vi "Abort.vi"(8 "error in (no error)":errorcluster, 11 "Parallell Test Runner in":refnum<class "Parallel Test Runner.lvclass">) -> (0 "error out":errorcluster)   [LabVIEW 2020, in "Parallel Test Runner.lvclass"]
uses:
  Parallel Test Runner.lvclass
  Parallel Test Runner.lvclass/Parallel Test Runner.ctl
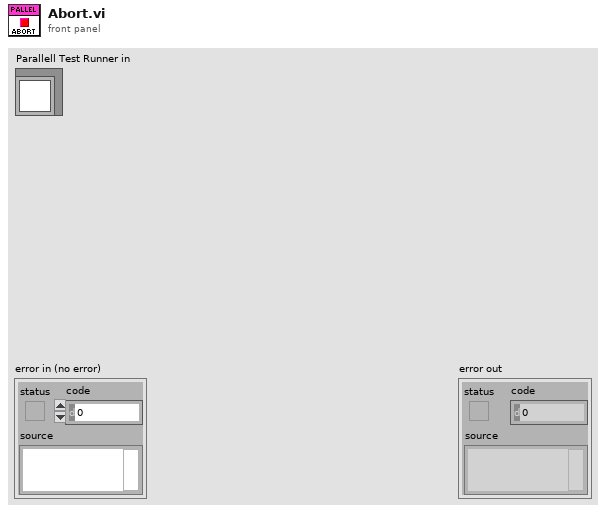
[diagram p1: front panel]
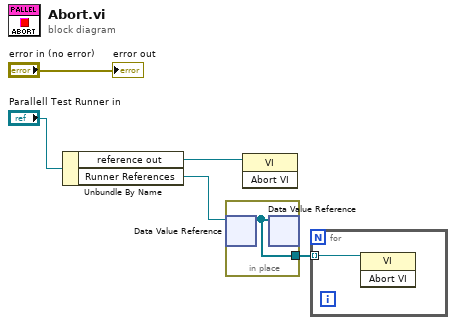
[diagram p0: block diagram]
diagram:
  n1 = Unbundle By Name("Parallell Test Runner in") -> ("reference out"=w3:refnum<vi>, "Runner References"=w2:refnum<data-value>)
  n2 = in-place {
    in-place-border: [w6] -> w1
    n3 = in-place-dvr #1(w2) -> (w6:refnum<vi>[])  [unwired: 1 out]
    n4 = in-place-dvr #1(w6) -> ()  [unwired: 2 out]
  }
  n5 = invoke class="VI" method="Abort VI"(reference=w3) -> ()  [unwired: 2 in, 3 out]
  n6 = for {
    tunnel: w1 -> [w7] mode=indexing
    n7 = invoke class="VI" method="Abort VI"(reference=w7) -> ()  [unwired: 2 in, 3 out]
  }
  "error out" <- "error in (no error)"
